vi "Manage Drive.vi"(7 "Min Drive Free Space (%)":dbl, 8 "error in":errorcluster, 11 "Data Folder":path=path "c:/data") -> (0 "error out":errorcluster, 2 "Drive Space Below Limit":bool, 3 "size (bytes)":i64)   [LabVIEW 2017]
panel:
  out "x*y":dbl
  out "free (bytes)":i64
  out "size (bytes) 2":i64
  out "All Files in Dir":path[](array[path])
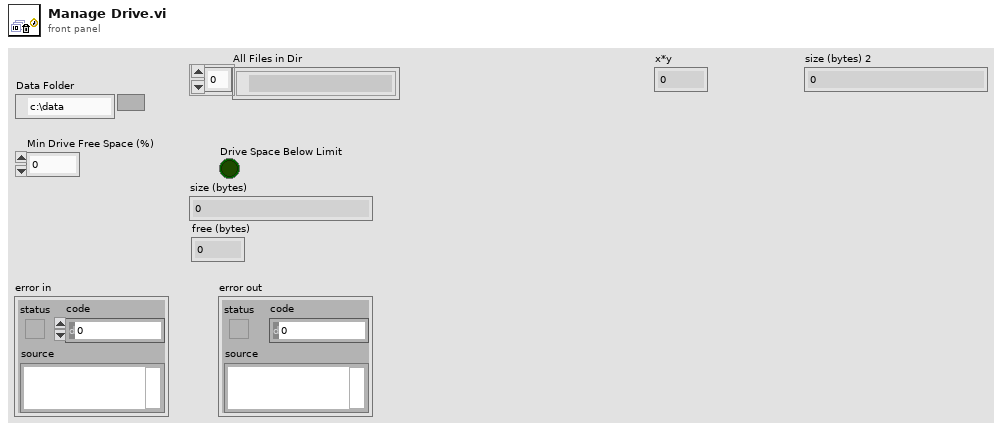
[diagram p1: front panel]
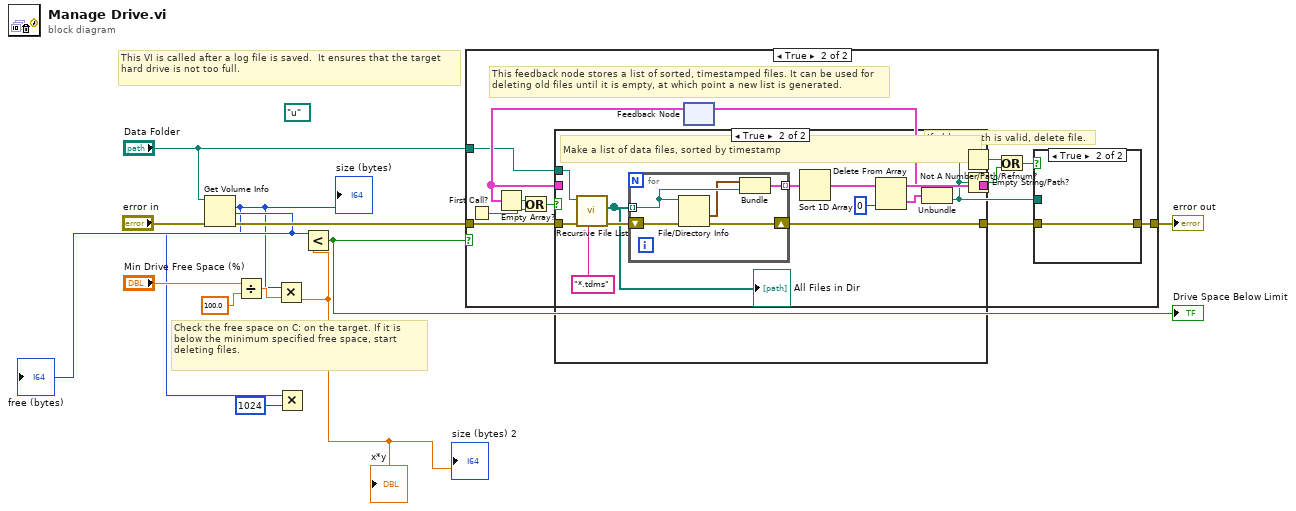
[diagram p0: block diagram]
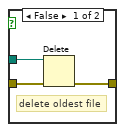
[diagram p3: hidden frame]
diagram:
  (unwired) path "u:/" ("AVI Path")
  # "Check the free space on C: on the target. If it is below the minimum specified free space, start deleting files."
  # "This VI is called after a log file is saved.  It ensures that the target hard drive is not too full."
  n1 = Get Volume Info(8:"error in", 11:"Data Folder") -> (0:w7:errorcluster, 1:w5:i64, 2:w3:i64)  [unwired: 3 out]
  "size (bytes)" <- w3
  "free (bytes)" <- w5
  n2 = Divide(x="Min Drive Free Space (%)", y=100.0) -> (x/y=w11:dbl)
  n3 = Multiply(x=w3, y=w11) -> (x*y=w1:dbl)
  "size (bytes) 2" <- w1
  "x*y" <- w1
  n4 = Multiply(x=w3, y=i64 1024) -> ()  [unwired: 1 out]
  n5 = Less?(x=w5, y=w1) -> (x < y?=w8:bool)
  "Drive Space Below Limit" <- w8
  n6 = case shown="True" w8 {
    tunnel: w7 -> [w13 w29]
    tunnel: [w13 w24] -> w6
    tunnel: "Data Folder" -> [_ w20]
    frame False {
      # "Free space is not below the minimum threshold.  Do nothing."
    }
    frame True {
      # "If oldest path is valid, delete file."
      # "This feedback node stores a list of sorted, timestamped files. It can be used for deleting old files until it is empty, at which point a new list is generated."
      n7 = First Call?() -> (First Call?: T/F=w27:bool)
      n8 = feedback #1() -> (w22:cluster{"last mod":timestamp, path}[])  [unwired: 1 out]
      n9 = Empty Array?(array=w22) -> (empty?=w21:bool)
      n10 = Or(x=w21, y=w27) -> (x .or. y?=w28:bool)
      n11 = case shown="True" w28 {
        tunnel: w29 -> [w35 w43]
        tunnel: [w35 w40] -> w23
        tunnel: [w34 w38] -> w26
        tunnel: w22 -> [w34 _]
        tunnel: w20 -> [_ w37]
        frame False {
          # "Current list of old files is non-empty.  Use it."
        }
        frame True {
          # "Make a list of data files, sorted by timestamp"
          n12 = call <vilib>:"Recursive File List.vi"("pattern"="*.tdms", "error in (no error)"=w43, "Folder Path"=w37) -> ("error out"=w41:errorcluster, "All Files in Dir"=w36:path[])  [unwired: 1 in, 6 out]
          "All Files in Dir" <- w36
          n13 = for {
            tunnel: w36 -> [w45] mode=indexing
            shift-right: [w47] -> w40
            shift-left: w41 -> [w48]
            tunnel: [w46] -> w39 mode=indexing
            n14 = File/Directory Info(path=w45, error in=w48) -> (last mod=w44:timestamp, error out=w47:errorcluster)  [unwired: 5 out]
            n15 = Bundle("last mod"=w44, w45) -> (w46:cluster{"last mod":timestamp, path})  [unwired: 1 out]
          }
          n16 = Sort 1D Array(array=w39) -> (sorted array=w38:cluster{"last mod":timestamp, path}[])
        }
      }
      n17 = Delete From Array(array=w26, index=0) -> (deleted portion=w18:cluster{"last mod":timestamp, path}, array with subset deleted=w25:cluster{"last mod":timestamp, path}[])  [unwired: 1 in]
      n18 = feedback-in #1(w25) -> ()
      n19 = Unbundle(w18) -> (w17:path)  [unwired: 1 out]
      n20 = Not A Number/Path/Refnum?(number/path/refnum=w17) -> (NaN/Path/Refnum?=w16:bool)
      n21 = Empty String/Path?(string/path=w17) -> (empty?=w15:bool)
      n22 = Or(x=w16, y=w15) -> (x .or. y?=w14:bool)
      n23 = case shown="True" w14 {
        tunnel: [w32 w33] -> w24
        tunnel: w23 -> [w31 w33]
        tunnel: w17 -> [w30 _]
        frame False {
          # "delete oldest file"
          n24 = Delete(path (use dialog)=w30, error in=w31) -> (error out=w32:errorcluster)  [unwired: 5 out]
        }
        frame True {
        }
      }
    }
  }
  "error out" <- w6
